vi "GLOBAL_odour_component_data.vi"() -> ()   [LabVIEW 2016]
panel:
  out "Odour component data":T1
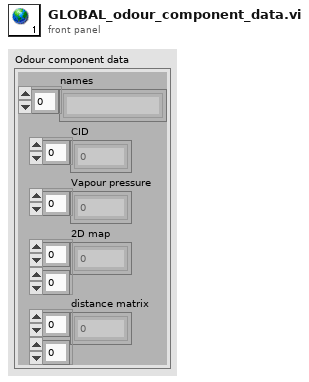
[diagram p1: front panel]
types:
  T1 = cluster{"names":string[], "CID":i32[], "Vapour pressure":dbl[], "2D map":dbl[][], "distance matrix":dbl[][]}
diagram:
